vi "PackageMessage.vi"(9 "Value":string, 10 "Name":string) -> (2 "Message":T1)   [LabVIEW 2014, in "Raspberry Pi Compatible Compiler for LabVIEW.lvlib" / "SimpleMessaging.lvlib"]
uses:
  SimpleMessaging.lvlib
  MessageTD.ctl
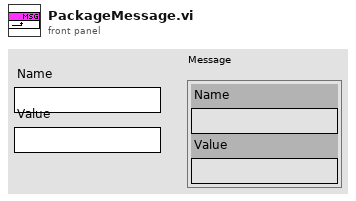
[diagram p1: front panel]
types:
  T1 = typedef "Raspberry Pi Compatible Compiler for LabVIEW.lvlib/SimpleMessaging.lvlib/MessageTD.ctl" = cluster{"Name":string, "Value":string}
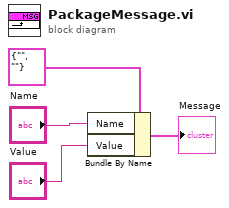
[diagram p0: block diagram]
diagram:
  n1 = Bundle By Name(cluster=T1 {"Name"="", "Value"=""} ("Message"), "Name"="Name", "Value"="Value") -> (→"Message":T1)
